vi "离线得到AD原码.vi"(7 "原始码":u8[](array[numeric]), 8 "错误输入":errorcluster caption="输出簇", 9 "原始码字节数":u32, 10 "通道索引":i32, 11 "文件句柄":i32) -> (0 "错误输出":errorcluster, 1 "数据个数":u32, 2 "AD原码":u16[](array[numeric]), 3 "文件句柄出":i32)   [LabVIEW 2011]
uses:
  dll/em9636.dll
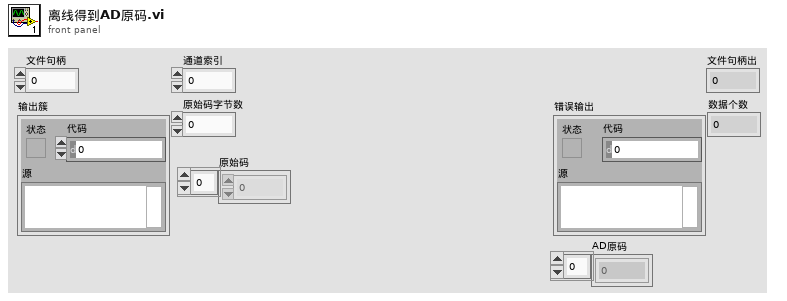
[diagram p1: front panel]
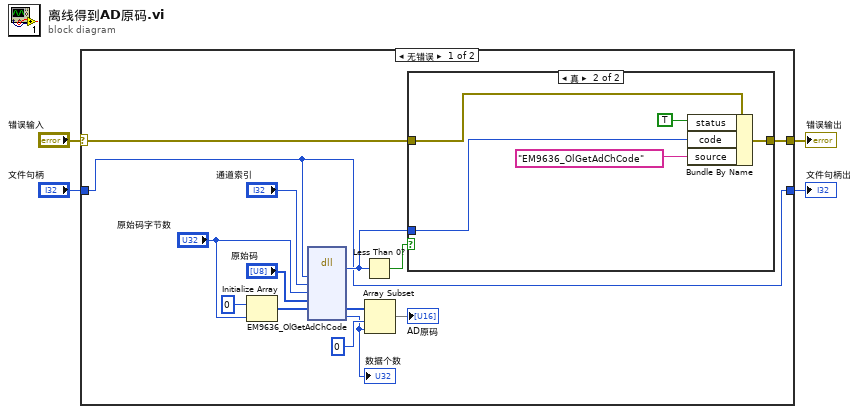
[diagram p0: block diagram]
diagram:
  n1 = case shown="无错误" "错误输入" {
    selector: "错误输入" -> [w14 w26]
    tunnel: [w16 w26] -> w3
    tunnel: "文件句柄" -> [w15 w25]
    tunnel: [w15 w25] -> w1
    frame No Error {
      n2 = Initialize Array(u16 0 ("元素"), "原始码字节数") -> (w9:u16[])
      n3 = dll-call lib="PTH1abs Eèµ éç LABVIEWæºVI(v2.0)EM9636BD)EM9636BDè°ç¨APIå½æ°æ¹æ³éè®¯ä¾ç¨EM9636labview8.5-1511048.5dll\nem9636.dll" fn="EM9636_OlGetAdChCode"("文件句柄"=w15, "通道索引"="通道索引", "原始码字节数"="原始码字节数", "原始码"="原始码", "AD原码"=w9) -> ("错误信息"=w17:i32, "AD原码"=w8:u16[], "原码个数"=w6:u32)  [unwired: 8 in, 2 out]
      "数据个数" <- w6
      n4 = Less Than 0?(x=w17) -> (x < 0?=w18:bool)
      n5 = Array Subset(array=w8, index=0 ("索引"), length=w6) -> (→"AD原码":u16[])
      n6 = case shown="真" w18 {
        tunnel: [w19 w22] -> w16
        tunnel: w14 -> [w19 w24]
        tunnel: w17 -> [_ w21]
        frame False {
        }
        frame True {
          n7 = Bundle By Name(cluster=w24, "status"=TRUE, "code"=w21, "source"="EM9636_OlGetAdChCode") -> (w22:errorcluster)
        }
      }
    }
    frame Error {
    }
  }
  "文件句柄出" <- w1
  "错误输出" <- w3
